vi "PlugIn AI.vi"(6 "String Value":string, 10 "Channel":T2, 11 "Menu":T1=enum."set avg_bits") -> ()   [LabVIEW 2019]
uses:
  <vilib>/Rock Robotics/SystemInterfaces/AI/FPGA_AIChannel.ctl
  AI Update Ops.ctl
panel:
  # "Don't place this VI anywhere\nin your API code. It needs to\nbe a dynamically loaded\nwrapper of the main global"
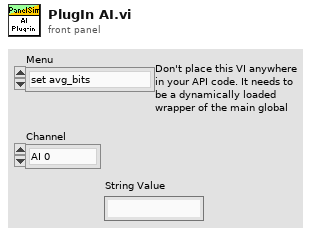
[diagram p1: front panel]
types:
  T1 = typedef "AI Update Ops.ctl" = enum16{"set init", "set avg_bits", "set oversample_bits", "set voltage", "set Accum_init", "set Accum_value", "set Accum_count", "set Accum_center", "set Accum_deadband", "get", "delete", "JSON update", "set  name", "transmit initial", "reset"}
  T2 = typedef "FPGA_AIChannel.ctl" = enum8{"AI 0", "AI 1", "AI 2", "AI 3", "AI MXP 0", "AI MXP 1", "AI MXP 2", "AI MXP 3", "Invalid"}
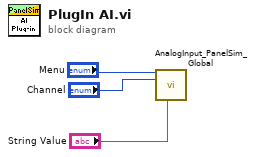
[diagram p0: block diagram]
diagram:
  n1 = call "AnalogInput_PanelSim_Global.vi"("menu"="Menu", "Channel"="Channel", "String Value"="String Value") -> ()  [unwired: 11 in, 2 out]
